vi "LogErrInfo.vi"(10 "location info":string, 11 "error in (no error)":errorcluster) -> (3 "error out":errorcluster)   [LabVIEW 2019, in "VsDebugLibrary.lvlib"]
uses:
  VsDebugLibrary.lvlib
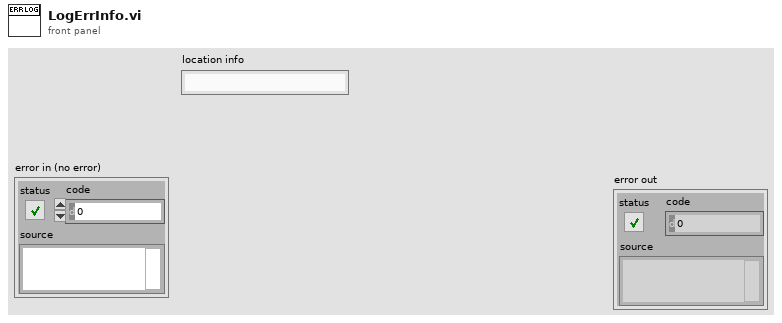
[diagram p1: front panel]
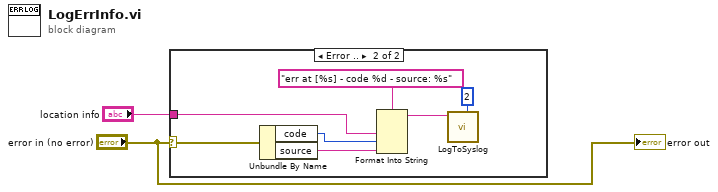
[diagram p0: block diagram]
diagram:
  n1 = case shown="Error .." "error in (no error)" {
    selector: "error in (no error)" -> [_ w9]
    tunnel: "location info" -> [_ w5]
    frame No Error {
    }
    frame Error {
      n2 = Unbundle By Name(w9) -> ("code"=w8:i32, "source"=w7:string)
      n3 = Format Into String(format string="err at [%s] - code %d - source: %s", w5, w8, w7) -> (resulting string=w4:string)  [unwired: 2 in, 1 out]
      n4 = call "LogToSyslog.vi"("call chain level (1)"=2, "message"=w4) -> ()  [unwired: 8 in, 2 out]
    }
  }
  "error out" <- "error in (no error)"
